vi "Test Name Forwarded to Wrapped Test Suite.vi"(8 "error in (no error)":errorcluster, 11 "Test Case In":refnum<class "Global Fixture Test.lvclass">) -> (0 "error out":errorcluster, 3 "Test Case Out":refnum<class "Global Fixture Test.lvclass">)   [LabVIEW 2020, in "Global Fixture Test.lvclass"]
uses:
  Global Fixture Test.lvclass
  C:/Program Files (x86)/National Instruments/LabVIEW 2020/vi.lib/Astemes/LUnit/Test Case.lvclass
  Global Fixture Test Double/Global Fixture Test Double.lvclass
  <vilib>/Astemes/LUnit/Test Case.lvclass/Test Case.ctl
  b6a9d788-022d-41aa-9c70-0533b6f2fd2e.vi
  <vilib>/Astemes/LUnit/Append Fail Result.vi
  <vilib>/Astemes/LUnit/Append Pass Result.vi
  <vilib>/Astemes/LUnit/Compare Variants.vi
  <vilib>/Astemes/LUnit/Describe Comparison.vi
  <vilib>/Astemes/LUnit/Run In UI.vi
  <vilib>/Utility/error.llb/Clear Errors.vi
  <vilib>/Astemes/LUnit/Describe Variant.vi
  <vilib>/Astemes/LUnit/Test Suite.lvclass
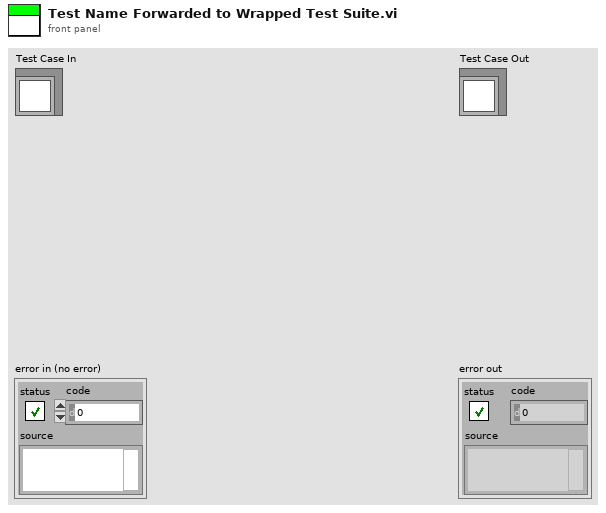
[diagram p1: front panel]
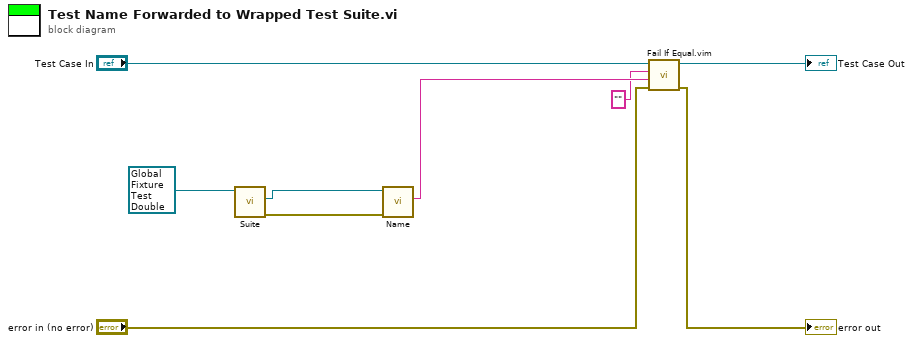
[diagram p0: block diagram]
diagram:
  n1 = call-dynamic "Suite.vi"("Global Fixture Test Case In"=refnum<class "Global Fixture Test Double.lvclass"> refnum ("Global Fixture Test Double.lvclass")) -> ("error out"=w3:errorcluster, "LUnit Test Suite Out"=w4:refnum<class "Test Suite.lvclass">)  [unwired: 8 in, 1 out]
  n2 = call-dynamic "Name.vi"("error in (no error)"=w3, "LUnit Test Suite in"=w4) -> ("Name"=w2:string)  [unwired: 7 in, 2 out]
  n3 = call "Fail If Equal.vim"("error in (no error)"="error in (no error)", "Actual"=w2, "Unexpected"="" ("Name"), "LUnit Test Case In"="Test Case In") -> ("error out"=→"error out":errorcluster, "LUnit Test Case Out"=→"Test Case Out":refnum<class "Global Fixture Test.lvclass">)  [unwired: 6 in]
